vi "Indexed Sort.vi"(2 "n":i32, 3 "A":sgl[](array[numeric])=[0.0, 0.0, 0.0, 0.0, 0.0, 0.0, 0.0, 0.0, 0.0, 0.0, 0.0, 0.0, 0.0, 0.0, 0.0, 0.0, 0.0, 0.0, 0.0, 0.0]) -> (0 "Index":i32[](array[numeric]), 1 "A Sorted":sgl[](array[numeric]))   [LabVIEW 2020]
uses:
  <vilib>/rvi/Emulation/niFpgaGetClockAttributes.vi
  <vilib>/rvi/Emulation/niFpgaSctlEmulationGetInTimedLoop.vi
  <vilib>/rvi/Emulation/niFpgaEmulationReportErrorSimple.vi
  <vilib>/rvi/Emulation/niFpgaCriticalErrorInLSC.vi
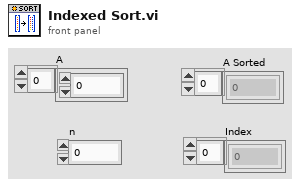
[diagram p1: front panel]
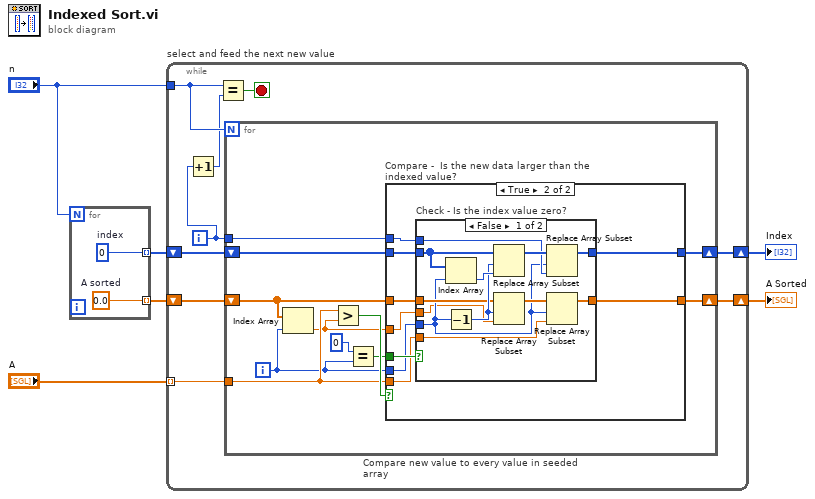
[diagram p0: block diagram]
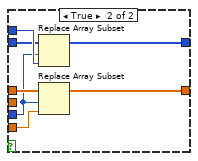
[diagram p3: hidden frame]
diagram:
  n1 = for {
    N: "n" -> [_]
    tunnel: [w8] -> w3 mode=indexing
    tunnel: [w7] -> w4 mode=indexing
    w7 = 0  # index
    w8 = sgl 0.0  # A sorted
  }
  n2 = while "select and feed the next new value" {
    shift-right: [w16] -> w5
    shift-left: w3 -> [w17]
    shift-right: [w15] -> w6
    shift-left: w4 -> [w14]
    tunnel: "n" -> [w11]
    tunnel: "A" -> [w12] mode=indexing
    i -> [w9]
    stop <- w13 stop-if-true
    n3 = Increment(x=w9) -> (x+1=w10:i32)
    n4 = Equal?(x=w11, y=w10) -> (x = y?=w13:bool)
    n5 = for "Compare new value to every value in seeded array" {
      N: w11 -> [_]
      tunnel: w12 -> [w26]
      shift-right: [w25] -> w16
      shift-left: w17 -> [w27]
      tunnel: w9 -> [w23]
      shift-right: [w21] -> w15
      shift-left: w14 -> [w22]
      i -> [w24]
      n6 = Index Array(array=w27, index=w24) -> (element=w18:sgl)
      n7 = Greater?(x=w26, y=w18) -> (0:w28:bool)
      n8 = Equal?(x=0, y=w24) -> (x = y?=w19:bool)
      n9 = case "Compare -  Is the new data larger than the indexed value?" shown="True" w28 {
        tunnel: w27 -> [w30 w38]
        tunnel: w19 -> [_ w39]
        tunnel: w26 -> [_ w37]
        tunnel: w24 -> [_ w36]
        tunnel: [w30 w35] -> w25
        tunnel: w23 -> [_ w34]
        tunnel: w22 -> [w29 w33]
        tunnel: [w29 w32] -> w21
        tunnel: w18 -> [_ w31]
        frame False {
        }
        frame True {
          n10 = case "Check - Is the index value zero?" shown="False" w39 {
            tunnel: w38 -> [w42 w58]
            tunnel: w37 -> [w50 w57]
            tunnel: w36 -> [w41 w52]
            tunnel: [w49 w56] -> w35
            tunnel: w34 -> [w44 w55]
            tunnel: w33 -> [w46 w54]
            tunnel: [w45 w53] -> w32
            tunnel: w31 -> [w40 _]
            frame False {
              n11 = Index Array(array=w46, index=w41) -> (element=w48:i32)
              n12 = Decrement(x=w41) -> (x-1=w43:i32)
              n13 = Replace Array Subset(array=w46, new element=w48, index=w43) -> (w47:i32[])
              n14 = Replace Array Subset(array=w42, new element=w40, index=w43) -> (w51:sgl[])
              n15 = Replace Array Subset(array=w47, new element=w44, index=w41) -> (w45:i32[])
              n16 = Replace Array Subset(array=w51, new element=w50, index=w41) -> (w49:sgl[])
            }
            frame True {
              n17 = Replace Array Subset(array=w54, new element=w55, index=w52) -> (w53:i32[])
              n18 = Replace Array Subset(array=w58, new element=w57, index=w52) -> (w56:sgl[])
            }
          }
        }
      }
    }
  }
  "Index" <- w6
  "A Sorted" <- w5
